vi "createEvents.vi"(8 "error in":errorcluster) -> (0 "error out":errorcluster, 1 "StopEvnts Out":T2, 2 "ElectEvnts Out":T1, 3 "FunctionalitiesEvnts Out":T3)   [LabVIEW 2016]
uses:
  ElectrometerController/controls/functionalitiesEvnts.ctl
  Electrometer/Modes.ctl
  ElectrometerController/controls/stopEvnts.ctl
  Electrometer/InternalEvents.ctl
  Electrometer/Electrometer.lvclass
  ElectrometerController/ElectrometerController.lvclass
panel:
  in  "ElectEvnts":T1
  in  "StopEvnts":T2
  in  "FunctionalitiesEvnts":T3
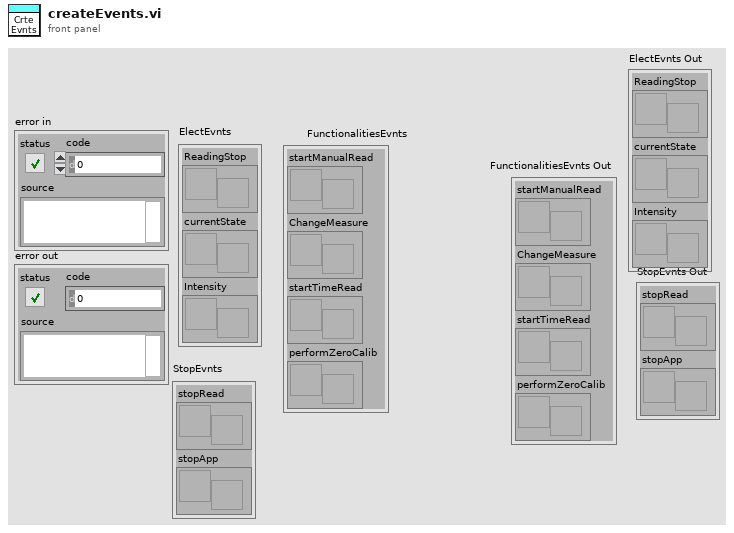
[diagram p1: front panel]
types:
  T1 = typedef "Electrometer.lvclass/InternalEvents.ctl" = cluster{"ReadingStop":refnum<user-event>, "currentState":refnum<user-event>, "Intensity":refnum<user-event>}
  T2 = typedef "ElectrometerController.lvclass/stopEvnts.ctl" = cluster{"stopRead":refnum<user-event>, "stopApp":refnum<user-event>}
  T3 = typedef "ElectrometerController.lvclass/functionalitiesEvnts.ctl" = cluster{"startManualRead":refnum<user-event>, "ChangeMeasure":refnum<user-event>, "startTimeRead":refnum<user-event>, "performZeroCalib":refnum<user-event>}
  T4 = cluster{"state":enum16{"Configuring", "Ready", "Reading"}}
  T5 = typedef "Electrometer.lvclass/Modes.ctl" = i32
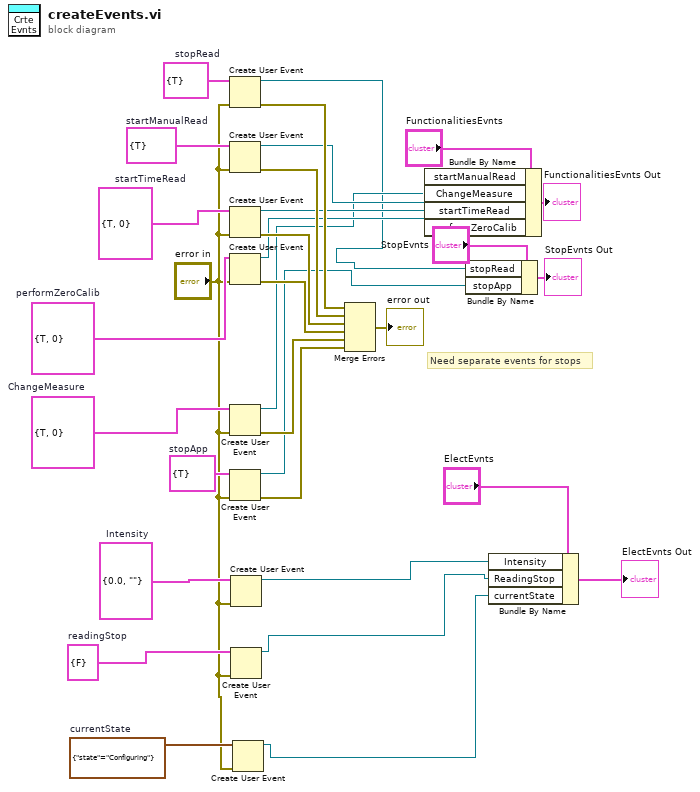
[diagram p0: block diagram]
diagram:
  w17 = T4 {"state"=enum."Configuring"}  # currentState
  w18 = cluster{"stop":bool} {"stop"=FALSE}  # readingStop
  w19 = cluster{"Intensity":dbl, "id":string} {"Intensity"=0.0, "id"=""}  # Intensity
  w28 = cluster{"DataSA":bool} {"DataSA"=TRUE}  # stopApp
  w27 = cluster{"DataCM":bool, "Mode":T5} {"DataCM"=TRUE, "Mode"=0}  # ChangeMeasure
  w29 = cluster{"DataZC":bool, "Mode":T5} {"DataZC"=TRUE, "Mode"=0}  # performZeroCalib
  w30 = cluster{"DataTR":bool, "Duration":i32} {"DataTR"=TRUE, "Duration"=0}  # startTimeRead
  w31 = cluster{"DataMR":bool} {"DataMR"=TRUE}  # startManualRead
  w32 = cluster{"DataSR":bool} {"DataSR"=TRUE}  # stopRead
  # "Need separate events for stops"
  n1 = Create User Event(user event datatype=w32, error in="error in") -> (user event=w8:refnum<user-event>, error out=w26:errorcluster)
  n2 = Create User Event(user event datatype=w31, error in="error in") -> (user event=w14:refnum<user-event>, error out=w25:errorcluster)
  n3 = Create User Event(user event datatype=w30, error in="error in") -> (user event=w13:refnum<user-event>, error out=w24:errorcluster)
  n4 = Create User Event(user event datatype=w29, error in="error in") -> (user event=w12:refnum<user-event>, error out=w22:errorcluster)
  n5 = Create User Event(user event datatype=w27, error in="error in") -> (user event=w11:refnum<user-event>, error out=w21:errorcluster)
  n6 = Create User Event(user event datatype=w28, error in="error in") -> (user event=w7:refnum<user-event>, error out=w20:errorcluster)
  n7 = Create User Event(user event datatype=w19, error in="error in") -> (user event=w1:refnum<user-event>)  [unwired: 1 out]
  n8 = Create User Event(user event datatype=w18, error in="error in") -> (user event=w4:refnum<user-event>)  [unwired: 1 out]
  n9 = Create User Event(user event datatype=w17, error in="error in") -> (user event=w3:refnum<user-event>)  [unwired: 1 out]
  n10 = Merge Errors(w26, w25, w24, w22, w21, w20) -> (→"error out":errorcluster)
  n11 = Bundle By Name(cluster="FunctionalitiesEvnts", "startManualRead"=w14, "ChangeMeasure"=w11, "startTimeRead"=w13, "performZeroCalib"=w12) -> (→"FunctionalitiesEvnts Out":T3)
  n12 = Bundle By Name(cluster="StopEvnts", "stopRead"=w8, "stopApp"=w7) -> (→"StopEvnts Out":T2)
  n13 = Bundle By Name(cluster="ElectEvnts", "Intensity"=w1, "ReadingStop"=w4, "currentState"=w3) -> (→"ElectEvnts Out":T1)
